vi "Check user abort.vi"(8 "error in (no error)":errorcluster, 11 "Common properties":T1={"Measurement status ref"=refnum, "TWM Status ref"=refnum, "Abort ref"=refnum, "Skip waiting ref"=refnum, "GNU Octave path"=path "C:/Program Files/GNU Octave/Octave-6.2.0/mingw64/bin", "TWM+QWTB path"=path "C:/Users/labina/Desktop/TWM-1.8.7.0-full/octprog", "lvlib path"=path "D:/martin/WAC/WACsw - github/control_software/Filter function meter/external libraries/GOLPI 0.7.3.1 source distribution LV 20.0 32 bit/lv_proc.dll", "TWM pipe"="\\\\.\\pipe\\TWM:server", "PJVS status ref"=refnum, "WAC path"=path ""}) -> (0 "error out":errorcluster)   [LabVIEW 2020]
doc: "Check if user abort happened. If so, create proper error."
uses:
  Type definitions/Common properties.ctl
  <vilib>/Utility/error.llb/Error Cluster From Error Code.vi
  <vilib>/ErrorRing/Error Ring.xnode
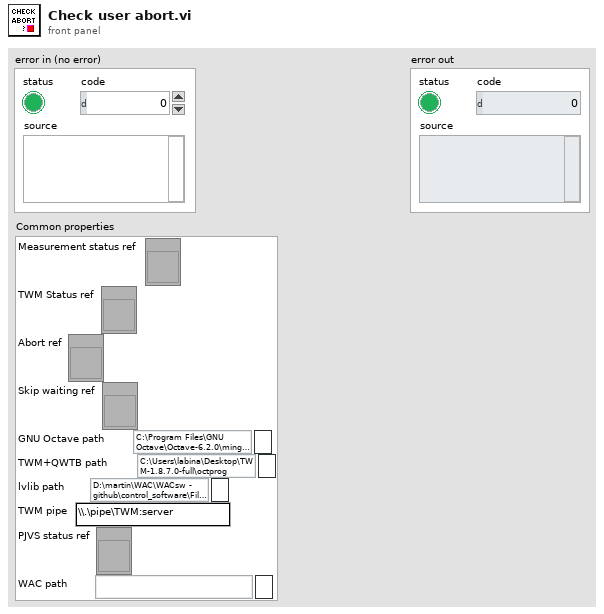
[diagram p1: front panel]
types:
  T1 = typedef "Common properties.ctl" = cluster{"Measurement status ref":refnum<vi>, "TWM Status ref":refnum<vi>, "Abort ref":refnum<vi>, "Skip waiting ref":refnum<vi>, "GNU Octave path":path, "TWM+QWTB path":path, "lvlib path":path, "TWM pipe":string, "PJVS status ref":refnum<vi>, "WAC path":path}
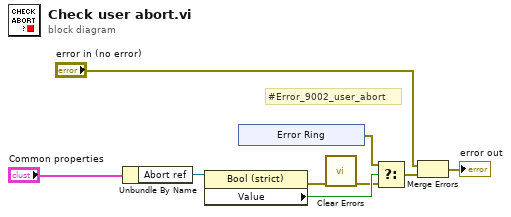
[diagram p0: block diagram]
diagram:
  # "#Error_9002_user_abort"
  n1 = Unbundle By Name("Common properties") -> ("Abort ref"=w8:refnum<vi>)
  n2 = property class="Bool (strict)"(reference=w8) -> (error out=w9:errorcluster, "Value"=w7:bool)  [unwired: 1 in, 1 out]
  n3 = xnode "Error Ring"() -> ("error out"=w6:errorcluster)
  n4 = call <vilib>:"Clear Errors.vi"("error in (no error)"=w9) -> ("error out"=w5:errorcluster)  [unwired: 5 in, 1 out]
  n5 = Select(t=w6, s=w7, f=w5) -> (s? t:f=w4:errorcluster)
  n6 = Merge Errors("error in (no error)", w4) -> (→"error out":errorcluster)
